vi "Bidirectional Quadrature Decoder with reset.vi"(9 "Reset":bool, 10 "B":bool, 11 "A":bool) -> (3 "Counter":i32)   [LabVIEW 2018]
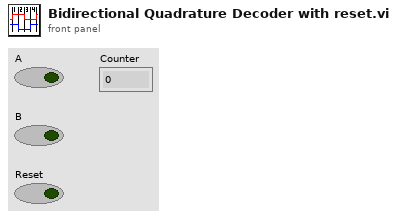
[diagram p1: front panel]
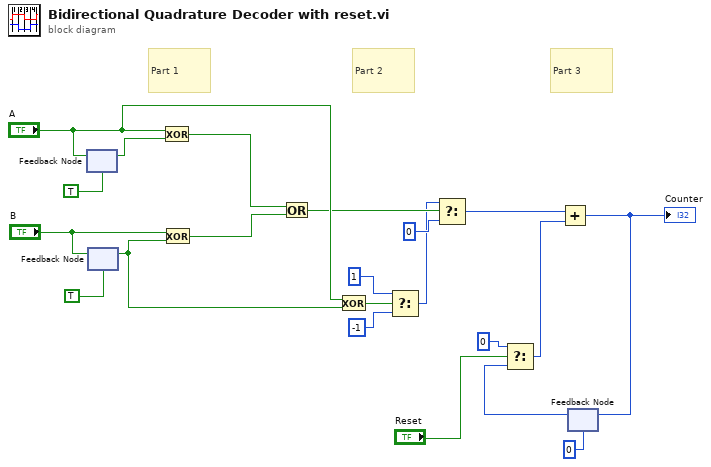
[diagram p0: block diagram]
diagram:
  # "Part 3"
  # "Part 2"
  # "Part 1"
  n1 = feedback #1(TRUE ("A")) -> (w16:bool)
  n2 = feedback-in #1("A") -> ()
  n3 = feedback #2(TRUE ("A")) -> (w18:bool)
  n4 = feedback-in #2("B") -> ()
  n5 = Exclusive Or(1:w16, 2:"A") -> (0:w14:bool)
  n6 = Exclusive Or(1:w18, 2:"B") -> (0:w9:bool)
  n7 = Or(x=w14, y=w9) -> (x .or. y?=w10:bool)
  n8 = Exclusive Or(1:w18, 2:"A") -> (0:w8:bool)
  n9 = Select(t=1, s=w8, f=-1) -> (s? t:f=w5:i32)
  n10 = Select(t=w5, s=w10, f=0) -> (s? t:f=w12:i32)
  n11 = feedback #3(0) -> (w19:i32)
  n12 = Select(t=0, s="Reset", f=w19) -> (s? t:f=w21:i32)
  n13 = Add(x=w12, y=w21) -> (x+y=w11:i32)
  "Counter" <- w11
  n14 = feedback-in #3(w11) -> ()
